vi "Write Data.vi"(8 "error in (no error)":errorcluster, 9 "Publication Time":timestamp, 10 "Value":variant, 11 "BooleanTextBinding in":refnum<class "BooleanTextBinding.lvclass">) -> (0 "error out":errorcluster, 3 "BooleanTextBinding out":refnum<class "BooleanTextBinding.lvclass">)   [LabVIEW 2015, in "Mediator.lvlib" / "BooleanTextBinding.lvclass"]
doc: "<License>\nCopyright © 2017 Composed Systems, LLC | All rights reserved\nwww.composed.io\n\nAuthor: Ethan Stern <ethan.stern@composed.io>\n\nThis software is provided \"AS IS\" WITHOUT WARRANTIES, either express or implied, AND IS FOR EDUCATIONAL PURPOSES ONLY.\n</License>"
uses:
  BooleanTextBinding.lvclass
  BooleanTextBinding.lvclass/BooleanTextBinding.ctl
  <vilib>/Utility/Data Type/NI_Data Type.lvlib
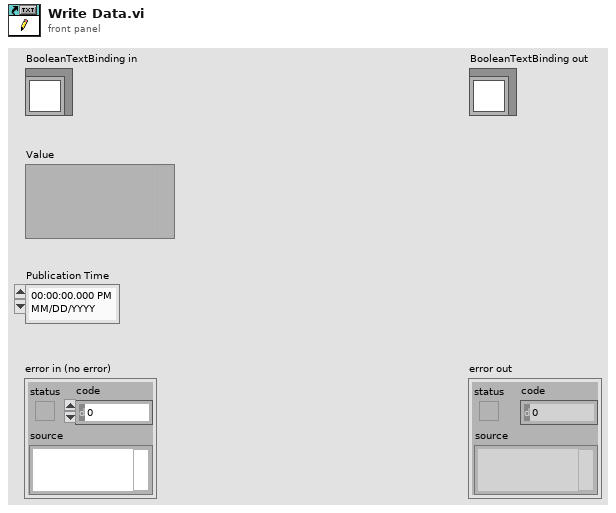
[diagram p1: front panel]
types:
  T1 = typedef "NI_Data Type.lvlib/Data Type.ctl" = enum8{"Invalid Type", "Void", "I8", "I16", "I32", "I64", "U8", "U16", "U32", "U64", "Single Float", "Double Float", "Extended Float", "Single Complex", "Double Complex", "Extended Complex", "Enum U8", "Enum U16", "Enum U32", "Enum U64", "Single Float With Unit", "Double Float With Unit", "Extended Float With Unit", "Single Complex with Unit", "Double Complex with Unit", "Extended Complex with Unit", "Boolean", "String", "Path", "Picture", "Tag", "Array", "Cluster", "Variant", "LV Variant", "Waveform", "Timestamp", "Digital Waveform", "Digital Data", "ExpressData", "Refnum", "External Data", "VI", "Poly VI", "LabVIEW Class Instance", "Fixed Point"}
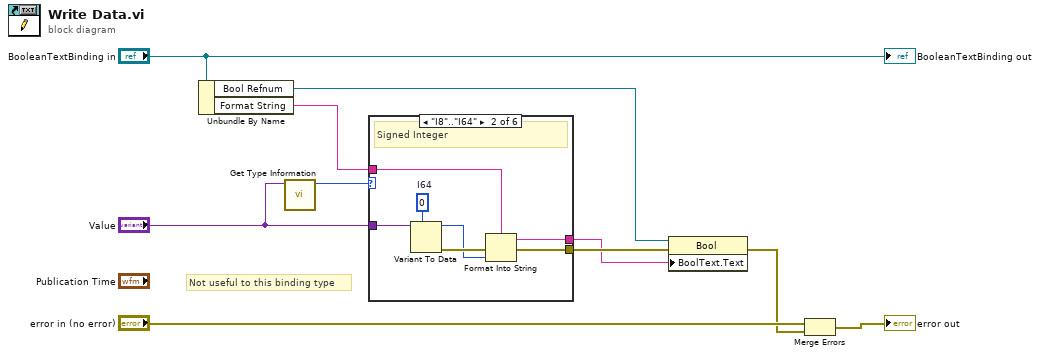
[diagram p0: block diagram]
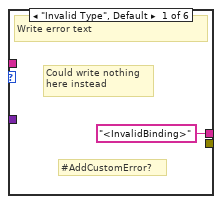
[diagram p2: hidden frame]
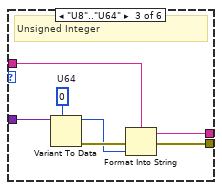
[diagram p3: hidden frame]
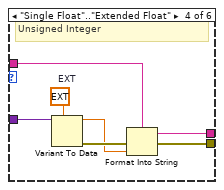
[diagram p4: hidden frame]
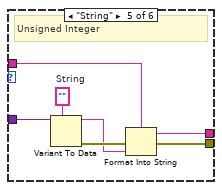
[diagram p5: hidden frame]
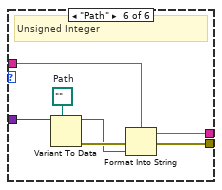
[diagram p6: hidden frame]
diagram:
  # "Not useful to this binding type"
  n1 = Unbundle By Name("BooleanTextBinding in") -> ("Bool Refnum"=w7:refnum<vi>, "Format String"=w5:string)
  n2 = call <vilib>:"Get Type Information.vi"("Variant"="Value") -> ("Type"=w1:T1)  [unwired: 6 in, 4 out]
  n3 = case shown="\"I8\"..\"I64\"" w1 {
    tunnel: "Value" -> [_ w18 w25 w32 w39 w46]
    tunnel: w5 -> [_ w17 w24 w31 w38 w45]
    tunnel: [_ w15 w22 w29 w36 w43] -> w4
    tunnel: ["<InvalidBinding>" w14 w21 w28 w35 w42] -> w3
    frame "Invalid Type", Default {
      # "#AddCustomError?"
      # "Could write nothing\nhere instead"
      # "Write error text"
    }
    frame "I8".."I64" {
      w12 = i64 0  # I64
      # "Signed Integer"
      n4 = Variant To Data(type=w12, Variant=w18) -> (data=w13:i64, error out=w16:errorcluster)  [unwired: 1 in]
      n5 = Format Into String(format string=w17, error in=w16, w13) -> (resulting string=w14:string, error out=w15:errorcluster)  [unwired: 1 in]
    }
    frame "U8".."U64" {
      w19 = u64 0  # U64
      # "Unsigned Integer"
      n6 = Variant To Data(type=w19, Variant=w25) -> (data=w20:u64, error out=w23:errorcluster)  [unwired: 1 in]
      n7 = Format Into String(format string=w24, error in=w23, w20) -> (resulting string=w21:string, error out=w22:errorcluster)  [unwired: 1 in]
    }
    frame "Single Float".."Extended Float" {
      w26 = ext 0.0  # EXT
      # "Unsigned Integer"
      n8 = Variant To Data(type=w26, Variant=w32) -> (data=w27:ext, error out=w30:errorcluster)  [unwired: 1 in]
      n9 = Format Into String(format string=w31, error in=w30, w27) -> (resulting string=w28:string, error out=w29:errorcluster)  [unwired: 1 in]
    }
    frame "String" {
      w33 = ""  # String
      # "Unsigned Integer"
      n10 = Variant To Data(type=w33, Variant=w39) -> (data=w34:string, error out=w37:errorcluster)  [unwired: 1 in]
      n11 = Format Into String(format string=w38, error in=w37, w34) -> (resulting string=w35:string, error out=w36:errorcluster)  [unwired: 1 in]
    }
    frame "Path" {
      w40 = path ""  # Path
      # "Unsigned Integer"
      n12 = Variant To Data(type=w40, Variant=w46) -> (data=w41:path, error out=w44:errorcluster)  [unwired: 1 in]
      n13 = Format Into String(format string=w45, error in=w44, w41) -> (resulting string=w42:string, error out=w43:errorcluster)  [unwired: 1 in]
    }
  }
  n14 = property class="Bool"(reference=w7, error in=w4, "BoolText.Text"=w3) -> (error out=w6:errorcluster)  [unwired: 1 out]
  n15 = Merge Errors("error in (no error)", w6) -> (→"error out":errorcluster)
  "BooleanTextBinding out" <- "BooleanTextBinding in"
